vi "test1.vi"() -> ()   [LabVIEW 2023]
panel:
  out "duty (%)":dbl
  in  "DUTY":dbl(knob) scale=0.0..100.0
  out "T (ms)":dbl
  in  "PERIOD":dbl(knob) scale=0.0..100.0
  out "OFF":bool
  out "ON":bool
  in  "ON/OFF":bool
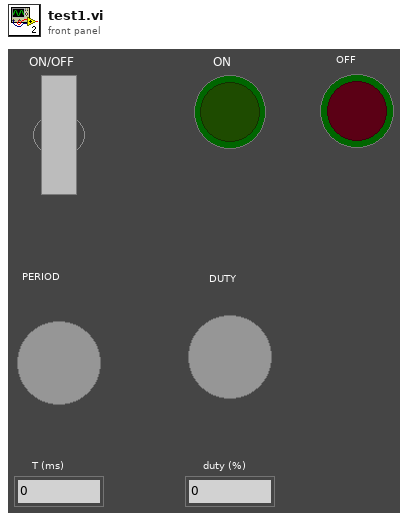
[diagram p1: front panel]
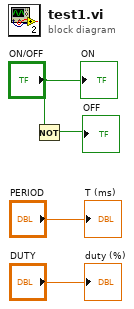
[diagram p0: block diagram]
diagram:
  n1 = Not(x="ON/OFF") -> (.not. x?=→"OFF":bool)
  "ON" <- "ON/OFF"
  "T (ms)" <- "PERIOD"
  "duty (%)" <- "DUTY"
